vi "Core Actor - DISPLAY - Message (String).vi"(8 "error in (no error)":errorcluster, 9 "Value":string, 11 "Child_2_Class in":refnum<class "Console_Class.lvclass">) -> (0 "error out":errorcluster, 3 "Child_2_Class out":refnum<class "Console_Class.lvclass">)   [LabVIEW 2023, in "Console_Actor.lvlib" / "Console_Class.lvclass"]
uses:
  Console_Class.lvclass
  Console_Class.lvclass/Console_Class.ctl
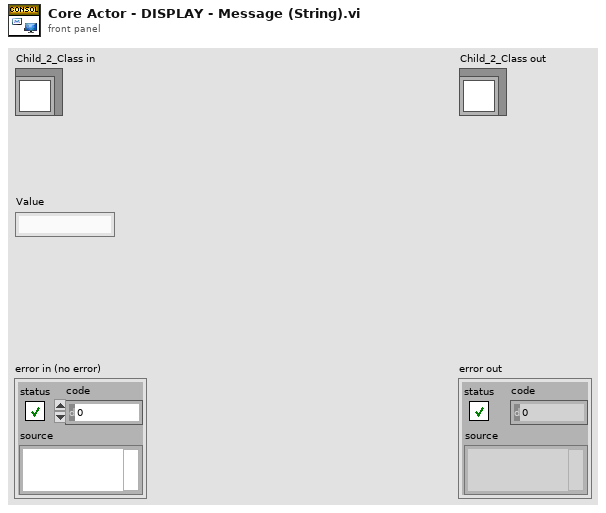
[diagram p1: front panel]
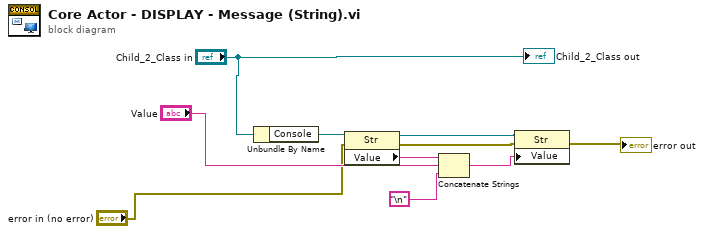
[diagram p0: block diagram]
diagram:
  n1 = Unbundle By Name("Child_2_Class in") -> ("Console"=w10:refnum<vi>)
  n2 = property class="Str"(reference=w10, error in="error in (no error)") -> (reference out=w8:refnum<vi>, error out=w7:errorcluster, "Value"=w9:string)
  n3 = Concatenate Strings(w9, "Value", "\n") -> (w6:string)
  n4 = property class="Str"(reference=w8, error in=w7, "Value"=w6) -> (error out=→"error out":errorcluster)  [unwired: 1 out]
  "Child_2_Class out" <- "Child_2_Class in"
